vi "Convert_to_Phys.vi"(1 "data in":u8[](array[numeric]), 2 "type descriptor":T1) -> (0 "value":dbl)   [LabVIEW 2014]
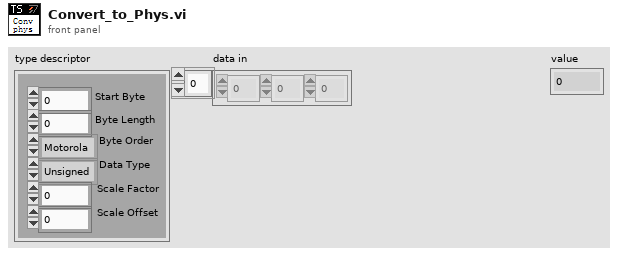
[diagram p1: front panel]
types:
  T1 = cluster{"Start Byte":i32, "Byte Length":i32, "Byte Order":enum16{"Motorola", "Intel"}, "Data Type":enum16{"Unsigned", "Signed", "Float"}, "Scale Factor":dbl, "Scale Offset":dbl}
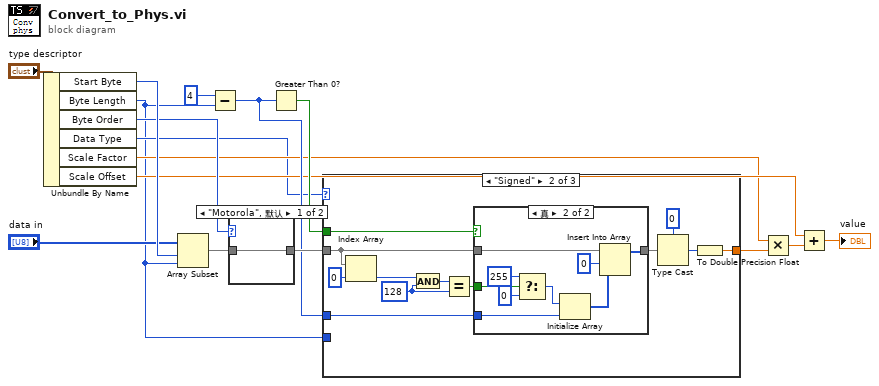
[diagram p0: block diagram]
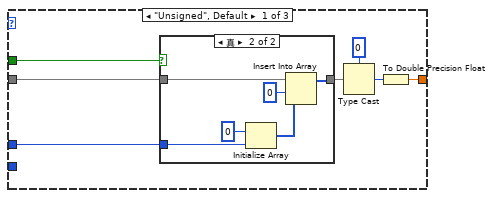
[diagram p2: hidden frame]
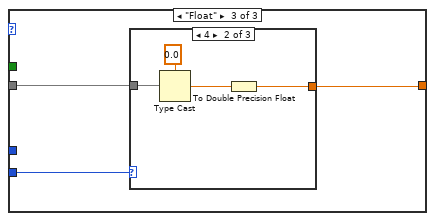
[diagram p5: hidden frame]
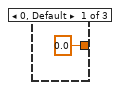
[diagram p6: hidden frame]
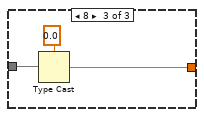
[diagram p7: hidden frame]
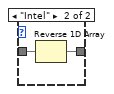
[diagram p8: hidden frame]
diagram:
  n1 = Unbundle By Name("type descriptor") -> ("Start Byte"=w15:i32, "Byte Length"=w1:i32, "Byte Order"=w12:enum16{"Motorola", "Intel"}, "Data Type"=w2:enum16{"Unsigned", "Signed", "Float"}, "Scale Factor"=w3:dbl, "Scale Offset"=w4:dbl)
  n2 = Array Subset(array="data in", index=w15, length=w1) -> (w13:u8[])
  n3 = Subtract(x=4, y=w1) -> (x-y=w5:i32)
  n4 = case shown="\"Motorola\", 默认" w12 {
    tunnel: w13 -> [w17 w19]
    tunnel: [w17 w18] -> w7
    frame "Motorola", Default {
    }
    frame "Intel" {
      n5 = Reverse 1D Array(array=w19) -> (reversed array=w18:u8[])
    }
  }
  n6 = Greater Than 0?(x=w5) -> (x > 0?=w6:bool)
  n7 = case shown="\"Signed\"" w2 {
    tunnel: [w20 w41 w56] -> w11
    tunnel: w7 -> [w25 w39 w57]
    tunnel: w6 -> [w24 w44 _]
    tunnel: w5 -> [w23 w40 _]
    tunnel: w1 -> [_ _ w58]
    frame "Unsigned", Default {
      n8 = case shown="真" w24 {
        tunnel: w25 -> [w27 w33]
        tunnel: [w27 w32] -> w22
        tunnel: w23 -> [_ w28]
        frame False {
        }
        frame True {
          n9 = Initialize Array(u8 0 ("element"), w28) -> (w30:u8[])
          n10 = Insert Into Array(array=w33, index=0, new element=w30) -> (w32:u8[])
        }
      }
      n11 = Type Cast(type=u32 0, x=w22) -> (*(type *) &x=w21:u32)
      n12 = To Double Precision Float(number=w21) -> (double precision float=w20:dbl)
    }
    frame "Signed" {
      w35 = u8 128 ("y")
      n13 = Index Array(array=w39, index=0) -> (element=w37:u8)
      n14 = And(x=w37, y=w35) -> (x .and. y?=w36:u8)
      n15 = Equal?(x=w36, y=w35) -> (x = y?=w34:bool)
      n16 = case shown="真" w44 {
        tunnel: w39 -> [w46 w55]
        tunnel: [w46 w54] -> w43
        tunnel: w40 -> [_ w51]
        tunnel: w34 -> [_ w50]
        frame False {
        }
        frame True {
          n17 = Select(t=u8 255, s=w50, f=u8 0) -> (s? t:f=w47:u8)
          n18 = Initialize Array(w47, w51) -> (w53:u8[])
          n19 = Insert Into Array(array=w55, index=0, new element=w53) -> (w54:u8[])
        }
      }
      n20 = Type Cast(type=0, x=w43) -> (*(type *) &x=w42:i32)
      n21 = To Double Precision Float(number=w42) -> (double precision float=w41:dbl)
    }
    frame "Float" {
      n22 = case shown="4" w58 {
        tunnel: w57 -> [_ w63 w66]
        tunnel: [0.0 w60 w64] -> w56
        frame 0, Default {
        }
        frame 4 {
          n23 = Type Cast(type=sgl 0.0, x=w63) -> (*(type *) &x=w61:sgl)
          n24 = To Double Precision Float(number=w61) -> (double precision float=w60:dbl)
        }
        frame 8 {
          n25 = Type Cast(type=0.0, x=w66) -> (*(type *) &x=w64:dbl)
        }
      }
    }
  }
  n26 = Multiply(x=w3, y=w11) -> (x*y=w10:dbl)
  n27 = Add(x=w4, y=w10) -> (x+y=→"value":dbl)
